vi "Delete.vi"(4 "Event #":i16=4, 5 "Sweep #":i16=4, 6 "Sweep trace (2D) In":cluster{"Ramp Pattern":dbl[], "X":dbl[]}[][](array[cluster]), 7 "Detected Event (1D) In":cluster{dbl[][]}[](array[cluster])) -> (2 "Sweep trace (2D) Out":cluster{"Ramp Pattern":dbl[], "X":dbl[]}[][](array[cluster]), 3 "Detected Event (1D) Out":cluster{dbl[][]}[](array[cluster]))   [LabVIEW 2017]
panel:
  out "삭제된 부분":dbl[][](array[numeric])
  in  "Whole trace":cluster{"Ramp Pattern":dbl[], "X":dbl[]}[](graph)
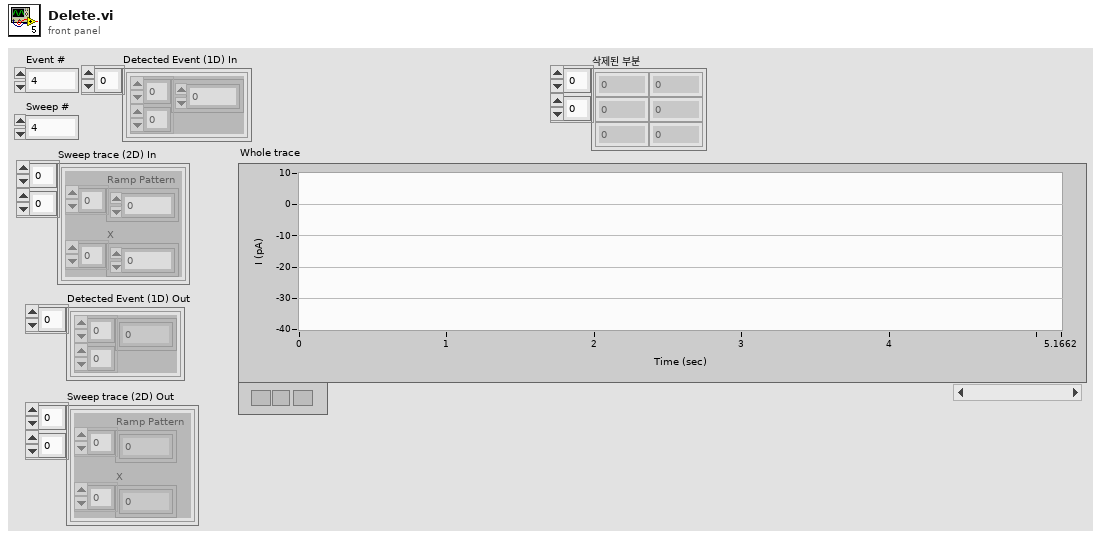
[diagram p1: front panel]
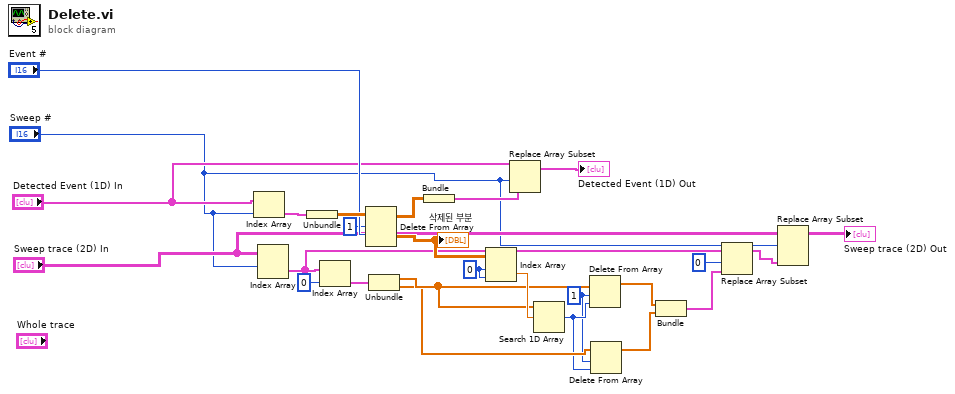
[diagram p0: block diagram]
diagram:
  w11 = 1 ("길이")
  w16 = 0 ("인덱스 (행)")
  n1 = Index Array(array="Detected Event (1D) In", index="Sweep #") -> (element=w26:cluster{dbl[][]})
  n2 = Index Array(array="Sweep trace (2D) In", index (row)="Sweep #") -> (element=w1:cluster{"Ramp Pattern":dbl[], "X":dbl[]}[])  [unwired: 1 in]
  n3 = Unbundle(w26) -> (w25:dbl[][])
  n4 = Index Array(array=w1, index=0 ("인덱스")) -> (element=w2:cluster{"Ramp Pattern":dbl[], "X":dbl[]})
  n5 = Delete From Array(array=w25, length=1 ("길이"), index (row)="Event #") -> (deleted portion=w17:dbl[][], array with subset deleted=w21:dbl[][])  [unwired: 1 in]
  "삭제된 부분" <- w17
  n6 = Unbundle(w2) -> ("Ramp Pattern"=w14:dbl[], "X"=w13:dbl[])
  n7 = Bundle(w21) -> (w20:cluster{dbl[][]})  [unwired: 1 in]
  n8 = Index Array(array=w17, index (row)=w16, index (col)=w16) -> (element=w15:dbl)
  n9 = Replace Array Subset(array="Detected Event (1D) In", new element=w20, index="Sweep #") -> (→"Detected Event (1D) Out":cluster{dbl[][]}[])
  n10 = Search 1D Array(1D array=w14, element=w15) -> (index of element=w12:i32)  [unwired: 1 in]
  n11 = Delete From Array(array=w14, length=w11, index=w12) -> (array with subset deleted=w10:dbl[])  [unwired: 1 out]
  n12 = Delete From Array(array=w13, length=w11, index=w12) -> (array with subset deleted=w9:dbl[])  [unwired: 1 out]
  n13 = Bundle("Ramp Pattern"=w10, "X"=w9) -> (w8:cluster{"Ramp Pattern":dbl[], "X":dbl[]})  [unwired: 1 in]
  n14 = Replace Array Subset(array=w1, new element=w8, index=0 ("인덱스")) -> (w5:cluster{"Ramp Pattern":dbl[], "X":dbl[]}[])
  n15 = Replace Array Subset(array="Sweep trace (2D) In", new element=w5, index (row)="Sweep #") -> (→"Sweep trace (2D) Out":cluster{"Ramp Pattern":dbl[], "X":dbl[]}[][])  [unwired: 1 in]
